vi "Mod2.vi"() -> ()   [LabVIEW 2014]
doc: "\"Discrete LED demo.vi\" -- Demonstrate a discrete LED connected to a digital output.\n\nInstructions:\n\n-- Click the 'enable blinker' button to toggle between blinking mode\nand static mode.\n-- In static mode, click the 'digital level' button to set the state of the\ndigital output.\n-- The 'digital output state' LED indicator shows the state of the\ndigital output (on = high, off = low)."
uses:
  <vilib>/myRIO/Common/Instrument Driver Framework/myRIO v1.0/UART/vis/myRIO v1.0 Close UART.vi
  <vilib>/Utility/error.llb/Error Cluster From Error Code.vi
  <vilib>/myRIO/Common/Instrument Driver Framework/myRIO v1.0/DIO/vis/myRIO v1.0 Write DIO.vi
  <vilib>/myRIO/Common/Instrument Driver Framework/Utilities/vis/FPGA Ref Manager.vi
  <vilib>/myRIO/Common/Instrument Driver Framework/myRIO v1.0/myRIO v1.0 Reset FPGA.vi
  <vilib>/myRIO/Common/Instrument Driver Framework/myRIO v1.0/IRQ/vis/myRIO v1.0 IRQ Info FGV.vi
  <vilib>/myRIO/Common/Instrument Driver Framework/myRIO v1.0/IRQ/vis/myRIO v1.0 Timer IRQ Info FGV.vi
  <vilib>/myRIO/Common/Instrument Driver Framework/myRIO v1.0/IRQ/vis/myRIO v1.0 ISR Agent.vi
  <vilib>/myRIO/Instrument Drivers/Utilities/Utilities.lvlib
  <vilib>/myRIO/Instrument Drivers/Onboard IO/DIO/DIO.lvlib
panel:
  in  "Enum":T1(ring)
  out "error out":errorcluster
  in  "error in (no error)":errorcluster
  in  "[ESC]":bool
  # "7-Segment LED demo"
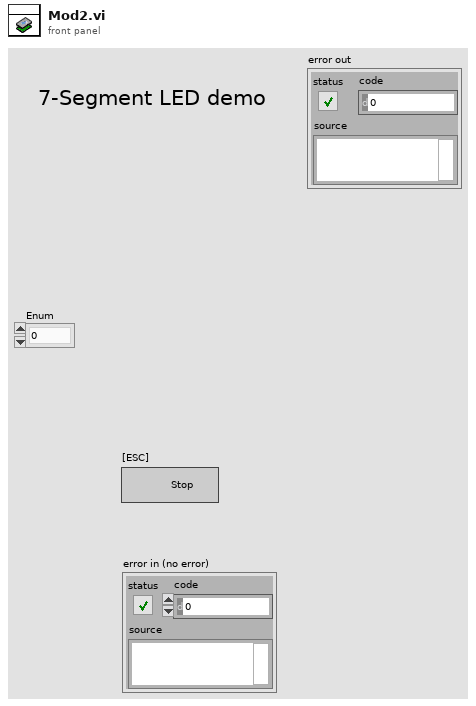
[diagram p1: front panel]
types:
  T1 = enum16{"0", "1", "2", "3", "4", "5", "6", "7", "8", "9", "A", "B", "C", "D", "E", "F"}
  T2 = typedef "DIO.lvlib/DIO Reference.ctl" = cluster{"myRIO Reference":T3, "DIO Channels List":T7}
  T3 = typedef "myRIO Generic Hardware Reference.ctl" = cluster{"myRIO Model":T4, "myRIO Hardware Reference":T5}
  T4 = typedef "Hardware Version Enum.ctl" = enum16{"Unknown", "myRIO-1900", "myRIO-1950"}
  T5 = typedef "myRIO v1.0 Reference.ctl" = cluster{"Generic FPGA Reference":T6, "Allow multiple opens":bool}
  T6 = typedef "Generic FPGA Reference.ctl" = refnum<k20>
  T7 = typedef "DIO Channels List.ctl" = T8[]
  T8 = typedef "DIO Channels Enum.ctl" = enum16{"Not Connected", "C/DIO0", "C/DIO1", "C/DIO2", "C/DIO3", "C/DIO4", "C/DIO5", "C/DIO6", "C/DIO7", "A/DIO0", "A/DIO1", "A/DIO2", "A/DIO3", "A/DIO4", "A/DIO5", "A/DIO6", "A/DIO7", "A/DIO8", "A/DIO9", "A/DIO10", "A/DIO11", "A/DIO12", "A/DIO13", "A/DIO14", "A/DIO15", "B/DIO0", "B/DIO1", "B/DIO2", "B/DIO3", "B/DIO4", "B/DIO5", "B/DIO6", "B/DIO7", "B/DIO8", "B/DIO9", "B/DIO10", "B/DIO11", "B/DIO12", "B/DIO13", "B/DIO14", "B/DIO15", "LED0", "LED1", "LED2", "LED3", "Button0"}
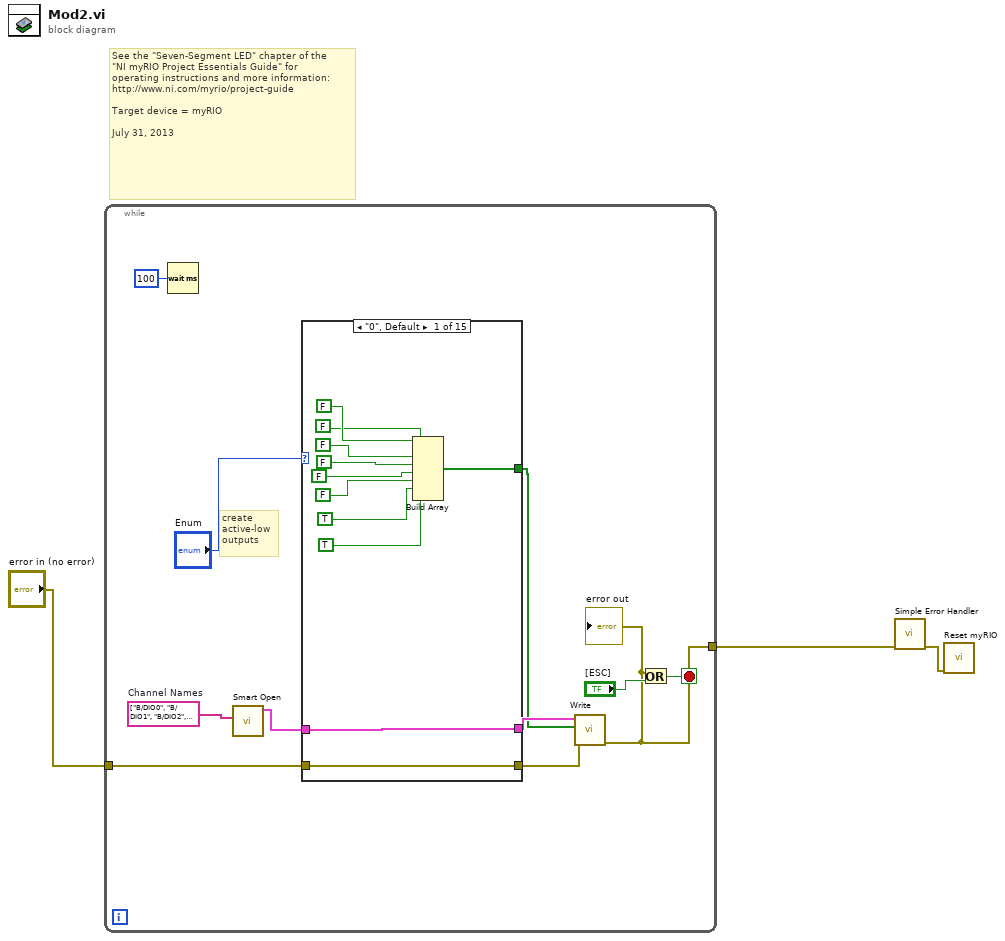
[diagram p0: block diagram]
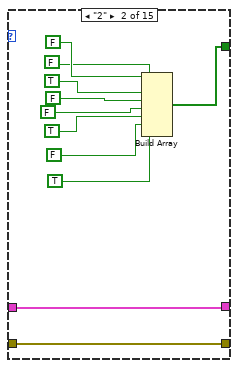
[diagram p2: hidden frame]
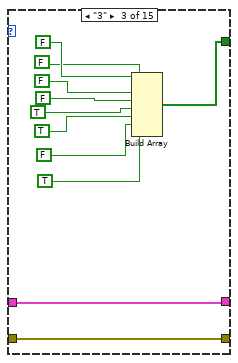
[diagram p3: hidden frame]
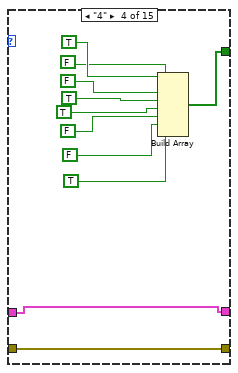
[diagram p4: hidden frame]
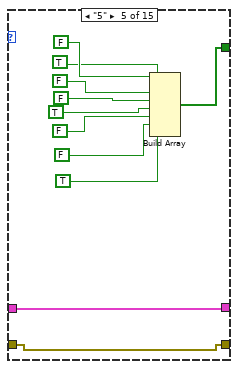
[diagram p5: hidden frame]
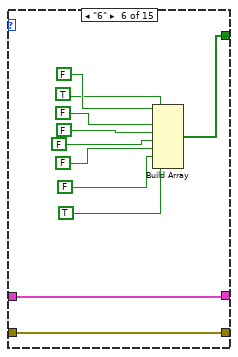
[diagram p6: hidden frame]
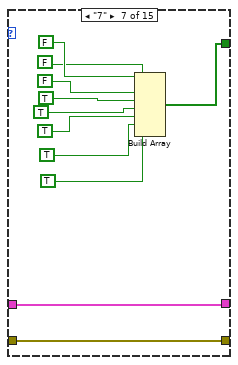
[diagram p7: hidden frame]
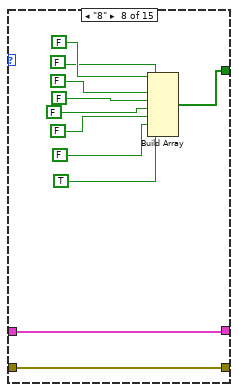
[diagram p8: hidden frame]
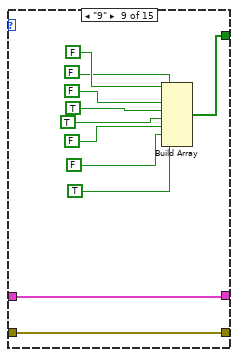
[diagram p9: hidden frame]
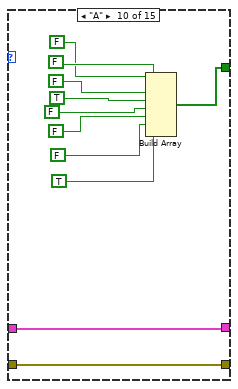
[diagram p10: hidden frame]
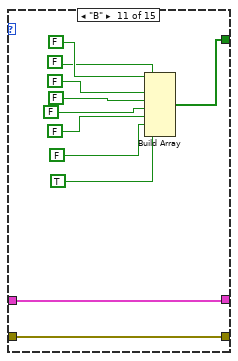
[diagram p11: hidden frame]
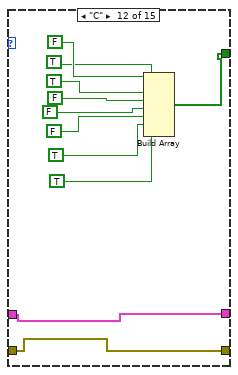
[diagram p12: hidden frame]
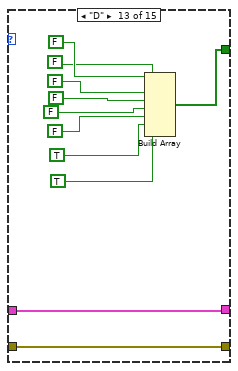
[diagram p13: hidden frame]
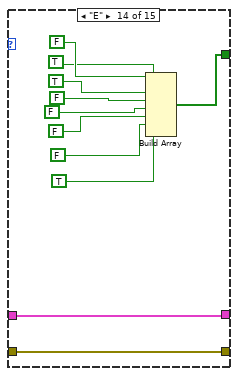
[diagram p14: hidden frame]
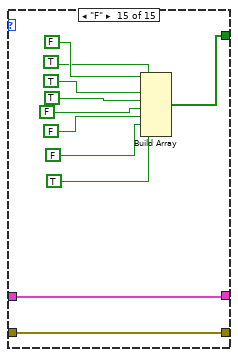
[diagram p15: hidden frame]
diagram:
  # "See the \"Seven-Segment LED\" chapter of the\n\"NI myRIO Project Essentials Guide\" for\noperating instructions and more information: \nhttp://www.ni.com/myrio/project-guide\n\nTarget device = myRIO\n\nJuly 31, 2013"
  n1 = while {
    tunnel: [w10] -> w2
    tunnel: "error in (no error)" -> [w7]
    stop <- w14 stop-if-true
    w11 = tag[] ["B/DIO0", "B/DIO1", "B/DIO2", "B/DIO3", "B/DIO4", "B/DIO5", "B/DIO6", "B/DIO7"]  # Channel Names
    # "create\nactive-low\noutputs"
    n2 = Wait (ms)(milliseconds to wait=u32 100) -> ()  [unwired: 1 out]
    n3 = call <vilib>:"Smart Open.vi"("Channel Names"=w11) -> ("DIO Ref Out"=w8:T2)  [unwired: 9 in, 1 out]
    n4 = case shown="\"0\", Default" "Enum" {
      tunnel: [w25 w27 w38 w49 w60 w71 w83 w102 w104 w116 w127 w138 w149 w161 w171] -> w9
      tunnel: w8 -> [w25 w27 w38 w49 w60 w71 w83 w102 w104 w116 w127 w138 w149 w161 w171]
      tunnel: w7 -> [w24 w26 w37 w48 w59 w72 w82 w101 w103 w115 w126 w137 w148 w160 w170]
      tunnel: [w24 w26 w37 w48 w59 w72 w82 w101 w103 w115 w126 w137 w148 w160 w170] -> w6
      tunnel: [w15 w28 w39 w50 w61 w70 w81 w92 w105 w117 w128 w139 w150 w158 w172] -> w5
      frame "0", Default {
        n5 = Build Array(FALSE, FALSE, FALSE, FALSE, FALSE, FALSE, TRUE, TRUE) -> (w15:bool[])
      }
      frame "2" {
        n6 = Build Array(FALSE, FALSE, TRUE, FALSE, FALSE, TRUE, FALSE, TRUE) -> (w28:bool[])
      }
      frame "3" {
        n7 = Build Array(FALSE, FALSE, FALSE, FALSE, TRUE, TRUE, FALSE, TRUE) -> (w39:bool[])
      }
      frame "4" {
        n8 = Build Array(TRUE, FALSE, FALSE, TRUE, TRUE, FALSE, FALSE, TRUE) -> (w50:bool[])
      }
      frame "5" {
        n9 = Build Array(FALSE, TRUE, FALSE, FALSE, TRUE, FALSE, FALSE, TRUE) -> (w61:bool[])
      }
      frame "6" {
        n10 = Build Array(FALSE, TRUE, FALSE, FALSE, FALSE, FALSE, FALSE, TRUE) -> (w70:bool[])
      }
      frame "7" {
        n11 = Build Array(FALSE, FALSE, FALSE, TRUE, TRUE, TRUE, TRUE, TRUE) -> (w81:bool[])
      }
      frame "8" {
        n12 = Build Array(FALSE, FALSE, FALSE, FALSE, FALSE, FALSE, FALSE, TRUE) -> (w92:bool[])
      }
      frame "9" {
        n13 = Build Array(FALSE, FALSE, FALSE, TRUE, TRUE, FALSE, FALSE, TRUE) -> (w105:bool[])
      }
      frame "A" {
        n14 = Build Array(FALSE, FALSE, FALSE, TRUE, FALSE, FALSE, FALSE, TRUE) -> (w117:bool[])
      }
      frame "B" {
        n15 = Build Array(FALSE, FALSE, FALSE, FALSE, FALSE, FALSE, FALSE, TRUE) -> (w128:bool[])
      }
      frame "C" {
        n16 = Build Array(FALSE, TRUE, TRUE, FALSE, FALSE, FALSE, TRUE, TRUE) -> (w139:bool[])
      }
      frame "D" {
        n17 = Build Array(FALSE, FALSE, FALSE, FALSE, FALSE, FALSE, TRUE, TRUE) -> (w150:bool[])
      }
      frame "E" {
        n18 = Build Array(FALSE, TRUE, TRUE, FALSE, FALSE, FALSE, FALSE, TRUE) -> (w158:bool[])
      }
      frame "F" {
        n19 = Build Array(FALSE, TRUE, TRUE, TRUE, FALSE, FALSE, FALSE, TRUE) -> (w172:bool[])
      }
    }
    n20 = call <vilib>:"Write.vi"("error in (no error)"=w6, "Values"=w5, "DIO Ref In"=w9) -> ("error out"=w10:errorcluster)  [unwired: 6 in, 1 out]
    "error out" <- w10
    n21 = Or(x=w10, y="[ESC]") -> (x .or. y?=w14:bool)
  }
  n22 = call <vilib>:"Simple Error Handler.vi"("error in (no error)"=w2) -> ("error out"=w3:errorcluster)  [unwired: 4 in, 4 out]
  n23 = call <vilib>:"Reset myRIO.vi"("error in (no error)"=w3) -> ()  [unwired: 10 in, 1 out]
